vi "Reply Enqueuer Name.vi"() -> (0 "Name":string)   [LabVIEW 2018, in "Scripting.lvlib"]
uses:
  Scripting.lvlib
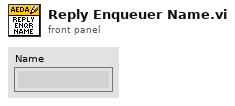
[diagram p1: front panel]
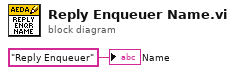
[diagram p0: block diagram]
diagram:
  "Name" <- "Reply Enqueuer" ("Label.Text")
